vi "MessdatenPeriode.vi"(7 "Quelle Indices \n(Erzeugen=1, Extern=0)":bool=TRUE, 8 "error in":errorcluster, 10 "Messdaten_Indices_Extern":dbl[](array[numeric]), 11 "Messdaten_Eingang(1-D)":dbl[](array[numeric])) -> (0 "error out":errorcluster, 1 "Anzahl Messwerte":i32, 2 "Indices_der_Schwellwerte":dbl[](array[numeric]), 3 "Messdaten_einer_periode":dbl[](array[numeric]), 4 "max Messwert":dbl, 6 "min Messwert":dbl)   [LabVIEW 2016]
doc: "Dem Vi wird ein periodisches Signal in Form eines 1D-Arrays übergeben. Als Ausgabe Array wird das periodische Signal auf eine Periode reduziert.\n\nAnmerkung:\nPerdiodisches Signal muss x-Achsensymetrisch sein.\nÜber boolschen Eingang, kann zwischen Arbeiten mit selber erzeugten Periodenindices oder extern erzeugten Periodenindices umgeschaltet werden."
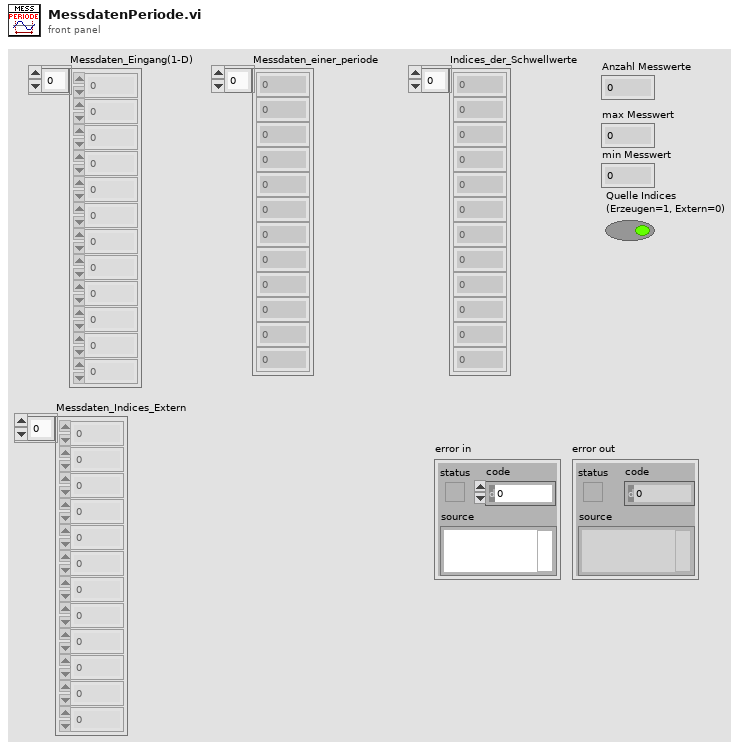
[diagram p1: front panel]
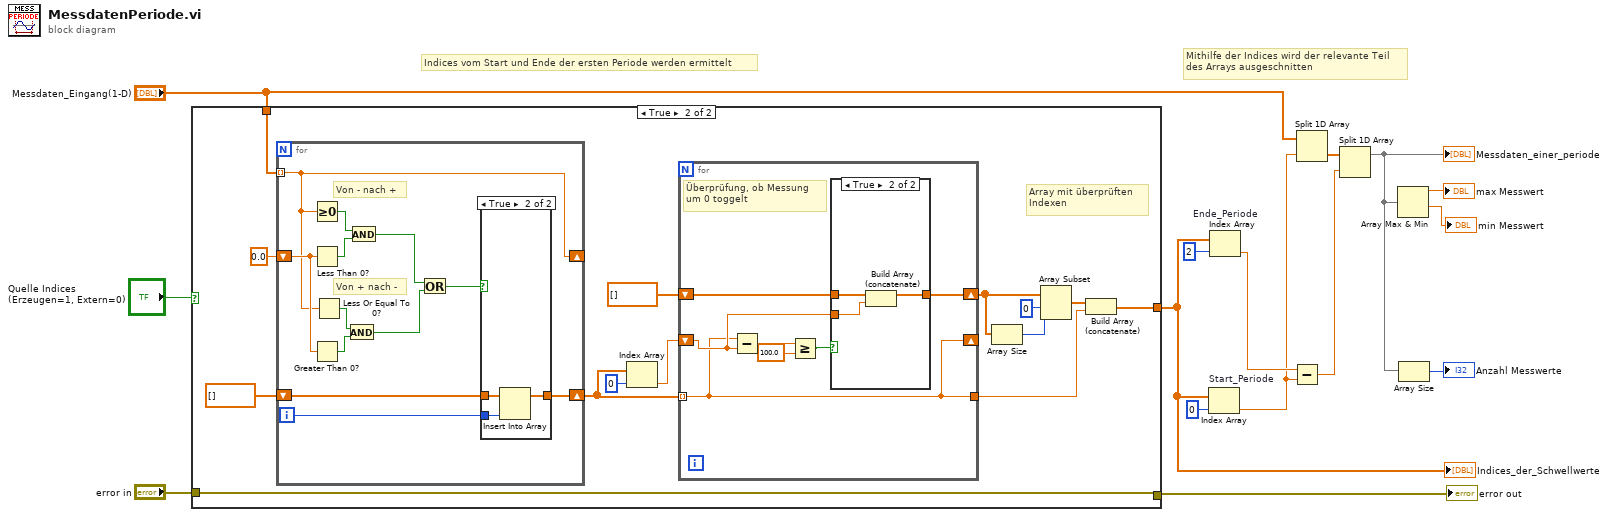
[diagram p0: block diagram]
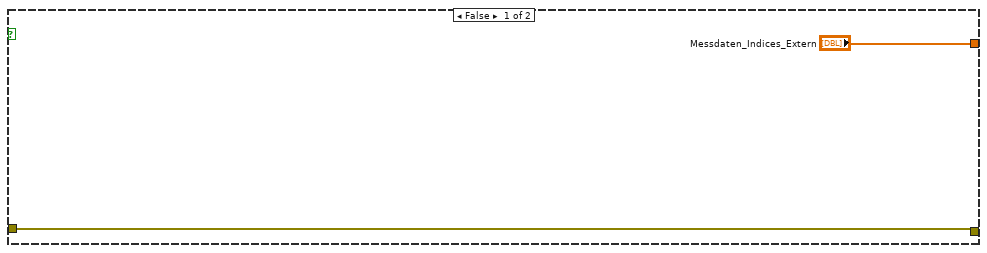
[diagram p2: hidden frame]
diagram:
  # "Mithilfe der Indices wird der relevante Teil\ndes Arrays ausgeschnitten"
  # "Indices vom Start und Ende der ersten Periode werden ermittelt"
  n1 = case shown="True" "Quelle Indices \n(Erzeugen=1, Extern=0)" {
    tunnel: "Messdaten_Eingang(1-D)" -> [_ w30]
    tunnel: [w17 w28] -> w4
    tunnel: "error in" -> [w17 w28]
    tunnel: ["Messdaten_Indices_Extern" w18] -> w2
    frame False {
    }
    frame True {
      # "Array mit überprüften \nIndexen"
      n2 = for {
        tunnel: w30 -> [w34] mode=indexing
        shift-right: [w34] -> _
        shift-left: 0.0 ("element") -> [w38]
        shift-right: [w41] -> w21
        shift-left: dbl[] [] -> [w40]
        i -> [w32]
        # "Von + nach -"
        # "Von - nach +"
        n3 = Greater Or Equal To 0?(x=w34) -> (x >= 0?=w43:bool)
        n4 = Less Than 0?(x=w38) -> (x < 0?=w42:bool)
        n5 = Greater Than 0?(x=w38) -> (x > 0?=w37:bool)
        n6 = Less Or Equal To 0?(x=w34) -> (x <= 0?=w36:bool)
        n7 = And(x=w36, y=w37) -> (x .and. y?=w35:bool)
        n8 = And(x=w43, y=w42) -> (x .and. y?=w39:bool)
        n9 = Or(x=w39, y=w35) -> (x .or. y?=w33:bool)
        n10 = case shown="True" w33 {
          tunnel: w32 -> [_ w45]
          tunnel: w40 -> [w44 w47]
          tunnel: [w44 w46] -> w41
          frame False {
          }
          frame True {
            n11 = Insert Into Array(array=w47, new element=w45) -> (w46:dbl[])  [unwired: 1 in]
          }
        }
      }
      n12 = Index Array(array=w21, index=0 ("Index")) -> (element=w24:dbl)
      n13 = for {
        tunnel: w21 -> [w48] mode=indexing
        tunnel: [w48] -> w19
        shift-right: [w48] -> _
        shift-left: w24 -> [w49]
        shift-right: [w53] -> w26
        shift-left: dbl[] [] -> [w54]
        # "Überprüfung, ob Messung\num 0 toggelt"
        n14 = Subtract(x=w48, y=w49) -> (x-y=w50:dbl)
        n15 = Greater Or Equal?(x=w50, y=100.0) -> (x >= y?=w52:bool)
        n16 = case shown="True" w52 {
          tunnel: w54 -> [w55 w58]
          tunnel: [w55 w57] -> w53
          tunnel: w49 -> [_ w56]
          frame False {
          }
          frame True {
            n17 = Build Array (concatenate)(w58, w56) -> (w57:dbl[])
          }
        }
      }
      n18 = Array Size(array=w26) -> (size(s)=w27:i32)
      n19 = Array Subset(array=w26, index=0 ("Index"), length=w27) -> (w20:dbl[])
      n20 = Build Array (concatenate)(w20, w19) -> (w18:dbl[])
    }
  }
  "Indices_der_Schwellwerte" <- w2
  "error out" <- w4
  n21 = Index Array "Start_Periode"(array=w2, index=0) -> (element=w12:dbl)
  n22 = Index Array "Ende_Periode"(array=w2, index=2) -> (element=w13:dbl)
  n23 = Subtract(x=w13, y=w12) -> (x-y=w11:dbl)
  n24 = Split 1D Array(array="Messdaten_Eingang(1-D)", index=w12) -> (second subarray=w14:dbl[])  [unwired: 1 out]
  n25 = Split 1D Array(array=w14, index=w11) -> (first subarray=w9:dbl[])  [unwired: 1 out]
  "Messdaten_einer_periode" <- w9
  n26 = Array Max & Min(array=w9) -> (max value=→"max Messwert":dbl, min value=→"min Messwert":dbl)  [unwired: 2 out]
  n27 = Array Size(array=w9) -> (size(s)=→"Anzahl Messwerte":i32)
